vi "Output 信息检测.vi"(9 "Output配置信息":string[][](table)=[["名称", "点位", "索引号"], ["三色灯红", "Y100", "0"], ["三色灯绿", "Y101", "1"], ["三色灯黄", "Y102", "2"], ["蜂鸣器", "Y103", "3"], ["上层真空电磁阀", "Y104", "4"], ["下层真空电磁阀", "Y105", "5"], ["传送抓手气缸", "Y106", "6"], ["上层产品定位气缸", "Y107", "7"], ["下层产品定位气缸", "Y110", "8"], ["起子1吸附真空", "Y111", "9"], ["起子2吸附真空", "Y112", "10"], ["起子3吸附真空", "Y113", "11"], ["起子4吸附真空", "Y114", "12"], ["起子1吹气电磁阀", "Y115", "13"], ["起子2吹气电磁阀", "Y116", "14"], ["起子3吹气电磁阀", "Y117", "15"], ["起子4吹气电磁阀", "Y120", "16"], ["光源", "Y121", "17"], ["Feed1指示灯", "Y122", "18"], ["Feed2指示灯", "Y123", "19"], ["Feed3指示灯", "Y124", "20"], ["Feed4指示灯", "Y125", "21"], ["上站取料完成反馈", "Y126", "22"], ["下站投料完成反馈", "Y127", "23"], ["上站给出请求信号", "Y130", "24"], ["下站给出答复信号", "Y131", "25"]], 11 "输出控制":T1) -> (2 "Output Error":string[](array[string]))   [LabVIEW 2017]
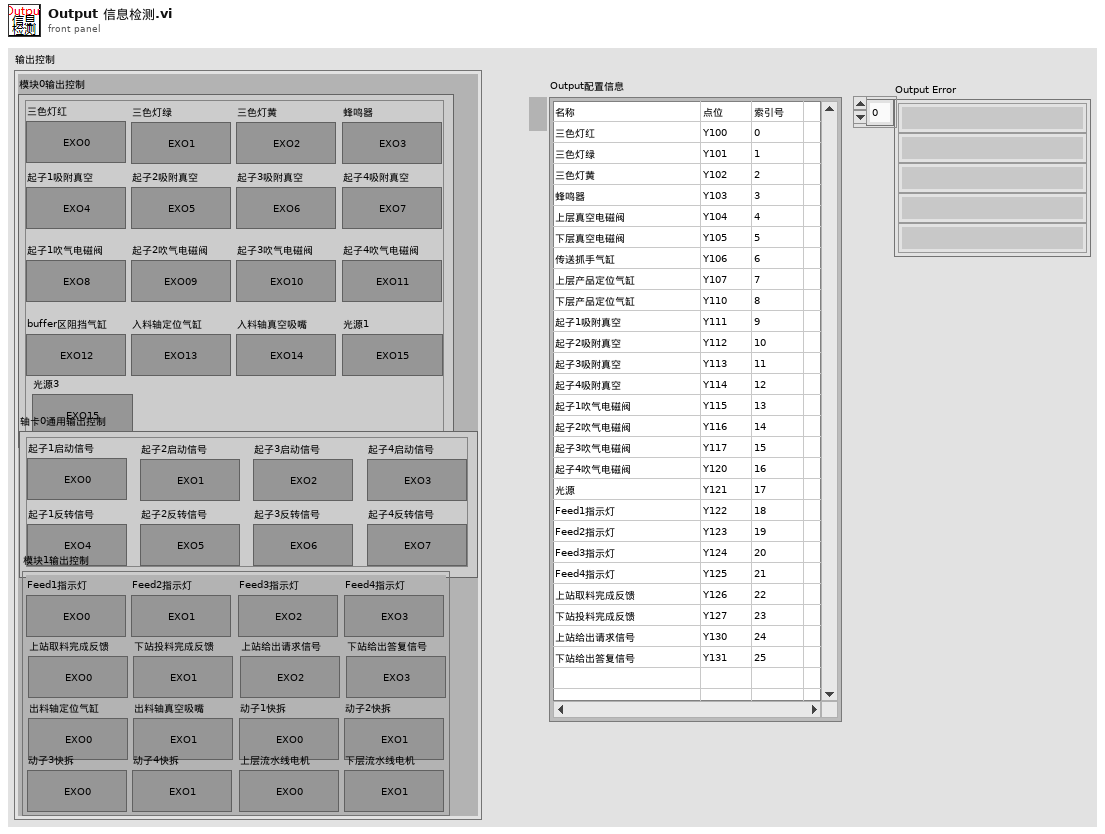
[diagram p1: front panel]
types:
  T1 = typedef "输出控制.ctl" = cluster{"模块0输出控制":T2, "轴卡0通用输出控制":T3, "模块1输出控制":T4}
  T2 = typedef "模块0输出控制.ctl" = cluster{"三色灯红":bool, "三色灯绿":bool, "三色灯黄":bool, "蜂鸣器":bool, "起子1吸附真空":bool, "起子2吸附真空":bool, "起子3吸附真空":bool, "起子4吸附真空":bool, "起子1吹气电磁阀":bool, "起子2吹气电磁阀":bool, "起子3吹气电磁阀":bool, "起子4吹气电磁阀":bool, "buffer区阻挡气缸":bool, "入料轴定位气缸":bool, "入料轴真空吸嘴":bool, "光源1":bool, "光源3":bool}
  T3 = typedef "轴卡0通用输出控制.ctl" = cluster{"起子1启动信号":bool, "起子2启动信号":bool, "起子3启动信号":bool, "起子4启动信号":bool, "起子1反转信号":bool, "起子2反转信号":bool, "起子3反转信号":bool, "起子4反转信号":bool}
  T4 = typedef "模块1输出控制.ctl" = cluster{"Feed1指示灯":bool, "Feed2指示灯":bool, "Feed3指示灯":bool, "Feed4指示灯":bool, "上站取料完成反馈":bool, "下站投料完成反馈":bool, "上站给出请求信号":bool, "下站给出答复信号":bool, "出料轴定位气缸":bool, "出料轴真空吸嘴":bool, "动子1快拆":bool, "动子2快拆":bool, "动子3快拆":bool, "动子4快拆":bool, "上层流水线电机":bool, "下层流水线电机":bool}
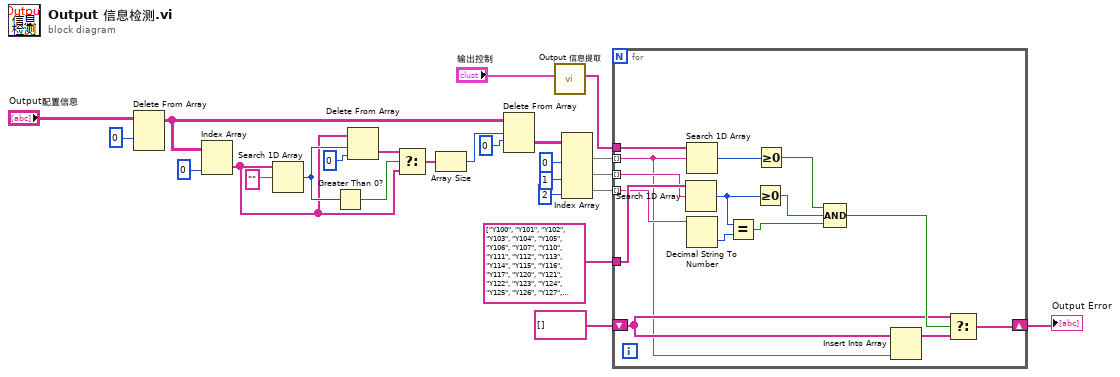
[diagram p0: block diagram]
diagram:
  n1 = Delete From Array(array="Output配置信息", index (row)=0 ("索引 (行)")) -> (array with subset deleted=w13:string[][])  [unwired: 2 in, 1 out]
  n2 = Index Array(array=w13, index (col)=0 ("禁用的索引 (列)")) -> (element=w16:string[])  [unwired: 1 in]
  n3 = Search 1D Array(1D array=w16, element="") -> (index of element=w20:i32)  [unwired: 1 in]
  n4 = Greater Than 0?(x=w20) -> (x > 0?=w21:bool)
  n5 = Delete From Array(array=w16, length=w20, index=0 ("索引")) -> (deleted portion=w18:string[])  [unwired: 1 out]
  n6 = Select(t=w18, s=w21, f=w16) -> (s? t:f=w15:string[])
  n7 = Array Size(array=w15) -> (size(s)=w17:i32)
  n8 = Delete From Array(array=w13, length=w17, index (row)=0 ("索引 (行)")) -> (deleted portion=w1:string[][])  [unwired: 1 in, 1 out]
  n9 = call "Output 信息提取.vi"("输出控制"="输出控制") -> ("Output 信息配置"=w3:string[])  [unwired: 10 in]
  n10 = Index Array(array=w1, index (col) #1=0 ("禁用的索引 (列)"), index (col) #2=1 ("禁用的索引 (列)"), index (col) #3=2 ("禁用的索引 (列)")) -> (element #1=w8:string[], element #2=w7:string[], element #3=w6:string[])  [unwired: 3 in]
  n11 = for {
    tunnel: w8 -> [w26] mode=indexing
    tunnel: w7 -> [w38] mode=indexing
    tunnel: w6 -> [w37] mode=indexing
    shift-right: [w28] -> w2
    shift-left: string[] [] -> [w30]
    tunnel: string[] ["Y100", "Y101", "Y102", "Y103", "Y104", "Y105", "Y106", "Y107", "Y110", "Y111", "Y112", "Y113", "Y114", "Y115", "Y116", "Y117", "Y120", "Y121", "Y122", "Y123", "Y124", "Y125", "Y126", "Y127", "Y130", "Y131", "Y132", "Y133", "Y134", "Y135", "Y136", "Y137", "Y140", "Y141", "Y142", "Y143", "Y144", "Y145", "Y146", "Y147", "Y150", "Y151", "Y152", "Y153", "Y154", "Y155", "Y156", "Y157", "Y160", "Y161", "Y162", "Y163", "Y164", "Y165", "Y166", "Y167", "Y170", "Y171", "Y172", "Y173", "Y174", "Y175", "Y176", "Y177"] ("子数组") -> [w39]
    tunnel: w3 -> [w27]
    n12 = Search 1D Array(1D array=w39, element=w38) -> (index of element=w36:i32)  [unwired: 1 in]
    n13 = Search 1D Array(1D array=w27, element=w26) -> (index of element=w40:i32)  [unwired: 1 in]
    n14 = Decimal String To Number(string=w37) -> (number=w35:i32)  [unwired: 2 in, 1 out]
    n15 = Equal?(x=w36, y=w35) -> (x = y?=w32:bool)
    n16 = Greater Or Equal To 0?(x=w36) -> (x >= 0?=w33:bool)
    n17 = Greater Or Equal To 0?(x=w40) -> (x >= 0?=w34:bool)
    n18 = Compound Arithmetic op=AND(w34, w33, w32) -> (w31:bool)
    n19 = Insert Into Array(array=w30, new element=w26) -> (w29:string[])  [unwired: 1 in]
    n20 = Select(t=w30, s=w31, f=w29) -> (s? t:f=w28:string[])
  }
  "Output Error" <- w2
